vi "Simulation - RT SO Plant FPGA PID.vi"() -> ()   [LabVIEW 2025]
doc: "This example demonstrates a process simulation for a tank level. The process has added noise, valve deadband, lag, and deadtime. A level controller adjusts the inflow to a tank. An on/off valve serves as a drain that you can click on to operate. This s-valve represents a change in the process loading. You also can switch this VI from automatic control to manual control."
uses:
  Process.ctl
  <vilib>/Utility/error.llb/Error Cluster From Error Code.vi
  <vilib>/rvi/errors/niLvFpgaAdjustHostInterfaceError.vi
  <vilib>/rvi/interface/nirviOpenFPGA/nirviOpenFPGA.xnode
  <vilib>/rvi/interface/nirviReadWriteControl/nirviReadWriteControl.xnode
  <vilib>/rvi/interface/nirviCloseFPGA/nirviCloseFPGA.xnode
  NiFpgaLv.dll
  <vilib>/rvi/interface/Simulation/niFpgaSimulationCallBeginRW.vi
  <vilib>/FPGAPlugInAG/Dynamic/niLvFpga_Close_Dynamic.vi
  FPGA Bitfiles/lvpidpyandso_FPGATarget_fpgapid_C9vj+qFiyHM.lvbitx
  PID_ValveController_CLIP/PID_ValveController/fpga pid.vi
  <vilib>/FPGAPlugInAG/cRIO-9040/niLvFpga_Open_cRIO-9040.vi
  <vilib>/rvi/interface/common/dynamic/niFpgaDynamicAddResources.vi
panel:
  in  "process":T1
  in  "Tab Control":enum32{"Introduction", "Operation"}(tab)=enum."Operation"
  in  "Setpoint":dbl(slide)=50.0 scale=0.0..100.0
  out "Flow sensor":bool
  in  "HV-101":bool
  out "tank level":dbl(slide) scale=0.0..100.0 scale format="%#.2g"
  out "Valve":bool
  out "Process Chart":T2(graph)
  in  "PID parameters":cluster{"Kc":dbl, "Ki":dbl, "Kd":dbl}={"Kc"=10.0, "Ki"=0.05, "Kd"=0.0} {"Kd" format="%#.6f"; "Ki" format="%#.4f"; "Kc" format="%#.4f"}
  in  "Stop":bool
  # "Tank Level Control"
  # "Overview: This example demonstrates a process simulation for a tank level.  The process has added noise, valve deadband, lag, and deadtime.  A level controller adjusts the inflow to a tank.  An on/off valve serves as a drain that you can click on to operate.  This s-valve represents a change in the process loading.  You also can switch this VI from automatic control to manual control.\nInstructions:\n1. Run the VI.\n2. Verify the PID controller in closed-loop to track the setpoint.\n3. Change the setpoint to another value and verify the controller tracking the new setpoint.\n4. Apply a disturbance to the system by switching the valve HV 102 (click on the valve symbol). You will see the controller recovering fro the change.\n5. Change PID gains and see if you can improve its performance without going unstable.\n6. Switch to manual mode and see if you can control the level by changing the Valve LVC 101.\n7. Click Stop to stop the VI."
  # "ISA Symbology: The diagram uses the ISA Symbology used for control"
  # "Loop 101"
  # "Level Controller at the control room"
  # "Level Transmitter on the field"
  # "Level Control Valve on the field"
  # "Hand Control Valve on the field"
  # "HV"
  # "102"
  # "LCV"
  # "101"
  # "LIC"
  # "101"
  # "LT"
  # "101"
  # "Slow Leak"
  # "Click to operate"
  # "HV"
  # "102"
  # "LCV"
  # "101"
  # "LIC"
  # "101"
  # "LT"
  # "101"
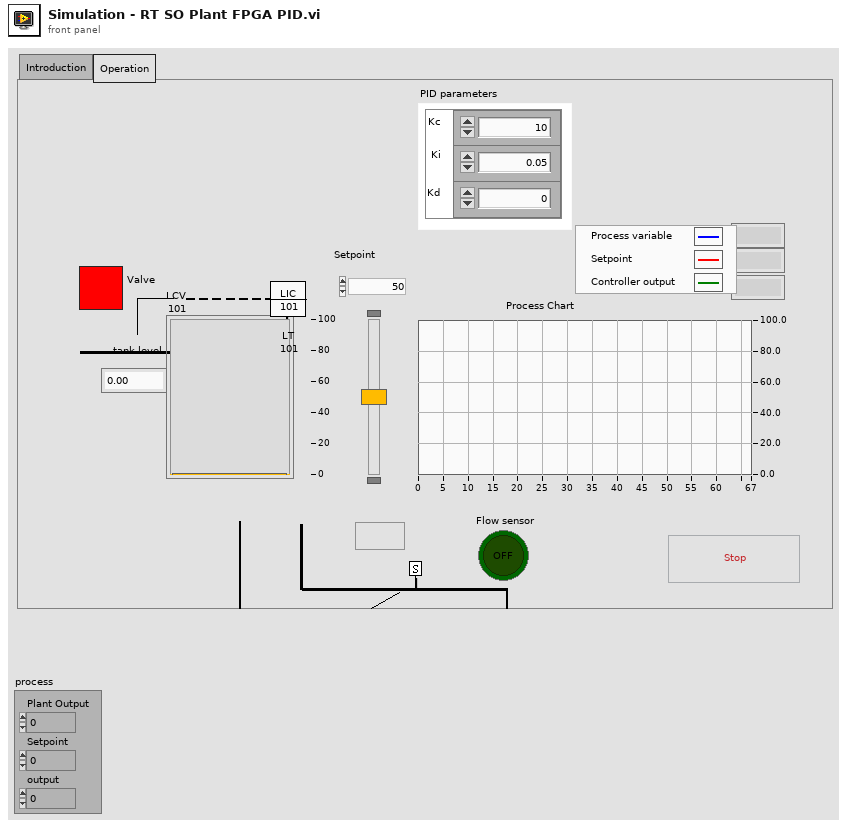
[diagram p1: front panel]
types:
  T1 = typedef "Process.ctl" = cluster{"Plant Output":dbl, "Setpoint":dbl, "output":dbl}
  T2 = cluster{"Plant Output":dbl, "Setpoint":dbl, "output":dbl}
  T3 = cluster{"static gain":dbl, "lag (s)":dbl, "deadtime (s)":dbl, "load":dbl, "deadband":dbl, "sensor noise":dbl, "initial PV":dbl, "plant noise":dbl}
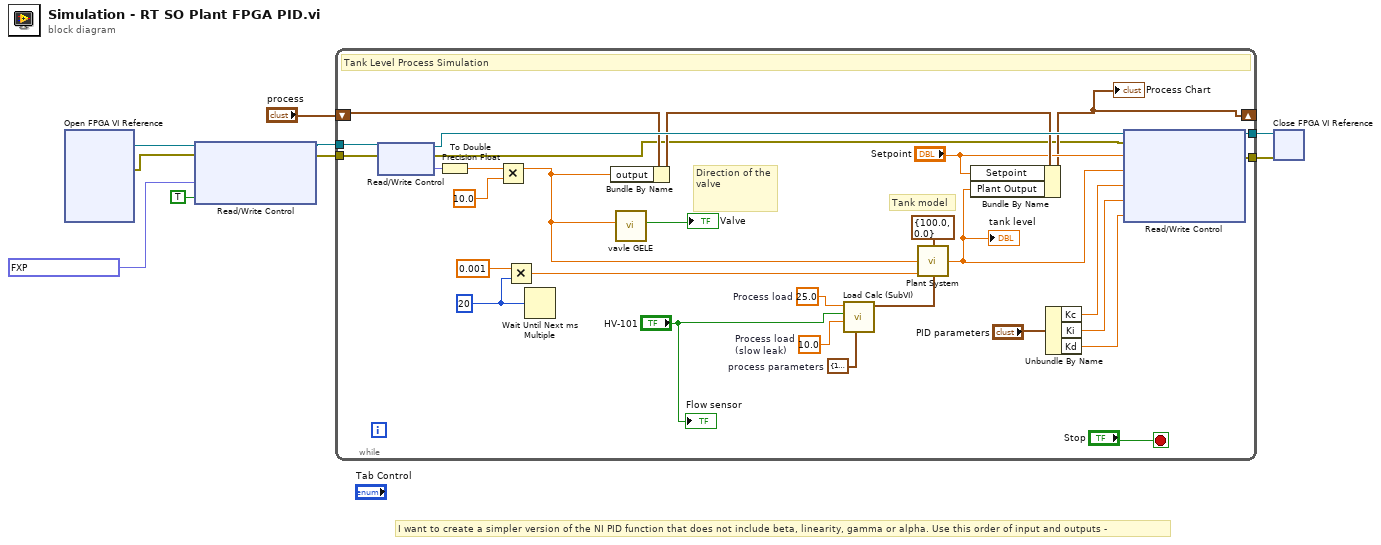
[diagram p0: block diagram]
diagram:
  # "I want to create a simpler version of the NI PID function that does not include beta, linearity, gamma or alpha. Use this order of input and outputs -"
  n1 = xnode "Open FPGA VI Reference"() -> ("FPGA VI Reference Out"=w9:refnum<k20>, "error out"=w8:errorcluster)  [unwired: 2 in]
  n2 = xnode "Read/Write Control"("FPGA VI Reference In"=w9, "error in"=w8, "KiCoeff"=fxp<+,32,16> 0.0099945068359375, "AutoMode"=TRUE) -> ("FPGA VI Reference Out"=w7:refnum<k20>, "error out"=w6:errorcluster)  [unwired: 1 in]
  n3 = while {
    tunnel: w7 -> [w30]
    tunnel: w6 -> [w29]
    tunnel: [w26] -> w5
    tunnel: [w25] -> w4
    shift-right: [w16] -> _
    shift-left: "process" -> [w24]
    stop <- "Stop" stop-if-true
    w38 = T3 {"static gain"=1.5, "lag (s)"=18.0, "deadtime (s)"=1.0, "load"=0.0, "deadband"=1.0, "sensor noise"=0.0, "initial PV"=0.0, "plant noise"=5.0}  # process parameters
    w35 = u32 20
    w32 = 25.0  # Process load
    w33 = 10.0  # Process load (slow leak)
    # "Tank model"
    # "Direction of the valve"
    # "Tank Level Process Simulation"
    n4 = xnode "Read/Write Control"("FPGA VI Reference In"=w30, "error in"=w29) -> ("FPGA VI Reference Out"=w27:refnum<k20>, "error out"=w13:errorcluster, "Output"=w28:fxp<+,32,16>)
    n5 = To Double Precision Float(number=w28) -> (double precision float=w22:dbl)
    n6 = Multiply(x=w22, y=10.0) -> (x*y=w11:dbl)
    n7 = Multiply(x=0.001, y=w35) -> (x*y=w34:dbl)
    n8 = Wait Until Next ms Multiple(millisecond multiple=w35) -> ()  [unwired: 1 out]
    n9 = Bundle By Name(cluster=w24, "output"=w11) -> (w23:T1)
    n10 = call "vavle GELE.vi"("output"=w11) -> ("T=Opening"=→"Valve":bool)  [unwired: 10 in]
    n11 = call "Load Calc (SubVI).vi"("process parameters in"=w38, "Leak load"=w33, "HV-101"="HV-101", "Process load"=w32) -> ("process parameters out"=w37:T3)  [unwired: 7 in]
    n12 = call "Plant System.vi"("output saturation range"=cluster{"output high":dbl, "output low":dbl} {"output high"=100.0, "output low"=0.0}, "Plant Input"=w11, "dt (s)"=w34, "process parameters"=w37) -> ("Plant Output"=w21:dbl)  [unwired: 11 in]
    "tank level" <- w21
    n13 = Bundle By Name(cluster=w23, "Setpoint"="Setpoint", "Plant Output"=w21) -> (w16:T1)
    "Process Chart" <- w16
    n14 = Unbundle By Name("PID parameters") -> ("Kc"=w18:dbl, "Ki"=w17:dbl, "Kd"=w14:dbl)
    n15 = xnode "Read/Write Control"("FPGA VI Reference In"=w27, "error in"=w13, "Setpoint"="Setpoint", "ProcessVariable"=w21, "ProportionalGainKc"=w18, "KiCoeff"=w17, "KdCoeff"=w14) -> ("FPGA VI Reference Out"=w26:refnum<k20>, "error out"=w25:errorcluster)
    "Flow sensor" <- "HV-101"
  }
  n16 = xnode "Close FPGA VI Reference"("FPGA VI Reference In"=w5, "error in"=w4) -> ()  [unwired: 1 out]
